vi "init.vi"(8 "error in (no error)":errorcluster, 11 "StiffnessMonitor in":refnum<class "StiffnessMonitor.lvclass">) -> (0 "error out":errorcluster, 3 "StiffnessMonitor out":refnum<class "StiffnessMonitor.lvclass">)   [LabVIEW 2013, in "StiffnessMonitor.lvclass"]
uses:
  StiffnessMonitor.lvclass
  Configuration/Stiffness Monitor.ctl
  StiffnessMonitor.lvclass/StiffnessMonitor.ctl
  ConfigurationThisComponent/ConfigurationThisComponent.lvclass
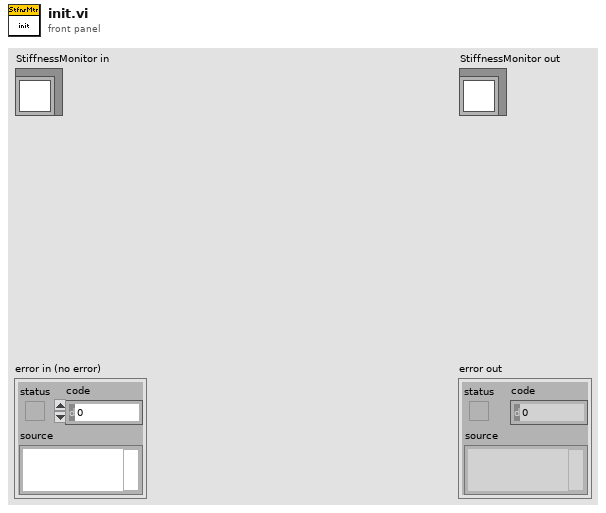
[diagram p1: front panel]
types:
  T1 = typedef "Stiffness Monitor.ctl" = cluster{"Stiffness Lower Limit":dbl[unit]}
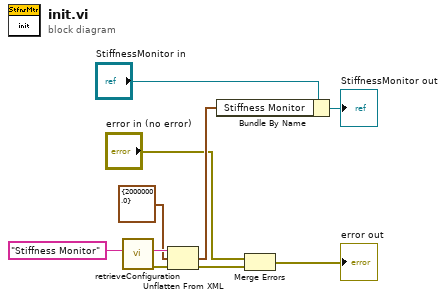
[diagram p0: block diagram]
diagram:
  n1 = call "retrieveConfiguration.vi"("configName"="Stiffness Monitor") -> ("error out"=w8:errorcluster, "xmlConfig"=w7:string)  [unwired: 8 in, 1 out]
  n2 = Unflatten From XML(xml string=w7, type=T1 {"Stiffness Lower Limit"=2000000.0} ("Stiffness Monitor"), error in (no error)=w8) -> (value=w3:T1, error out=w10:errorcluster)
  n3 = Bundle By Name(cluster="StiffnessMonitor in", "Stiffness Monitor"=w3) -> (→"StiffnessMonitor out":refnum<class "StiffnessMonitor.lvclass">)
  n4 = Merge Errors("error in (no error)", w10) -> (→"error out":errorcluster)
